vi "Multiple U3 Efunction Loop Example.vi"() -> (0 "error out 1":errorcluster)   [LabVIEW 2021]
panel:
  out "FIO5 State In 2":bool
  in  "DAC0 Voltage 2":dbl format="%.3f"
  in  "FIO4 State Out 2":bool
  out "Error Message 2":string
  out "error out 2":errorcluster
  out "AIN0 Voltage 2":dbl format="%.6f"
  in  "stop":bool
  in  "Interval (ms)":u32=500
  out "FIO5 State In 1":bool
  in  "DAC0 Voltage 1":dbl format="%.3f"
  in  "FIO4 State Out 1":bool
  out "Error Message 1":string
  out "AIN0 Voltage 1":dbl format="%.6f"
  # "U3 with LocalID=1:  Sets DAC0, sets FIO4,\nreads AIN0, and reads FIO5."
  # "U3 with LocalID=2:  Sets DAC0, sets FIO4,\nreads AIN0, and reads FIO5."
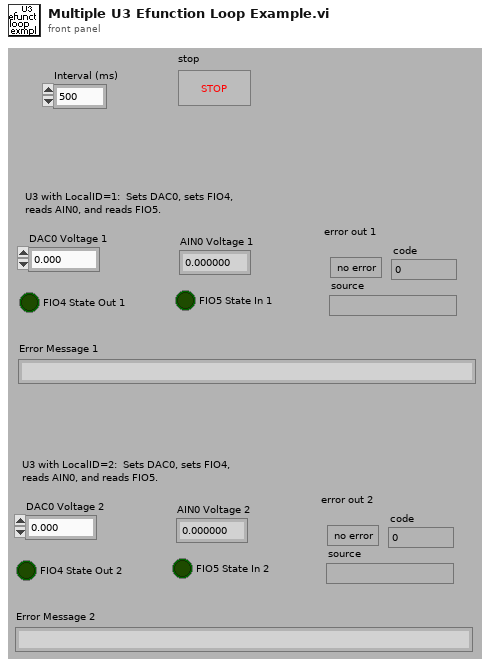
[diagram p1: front panel]
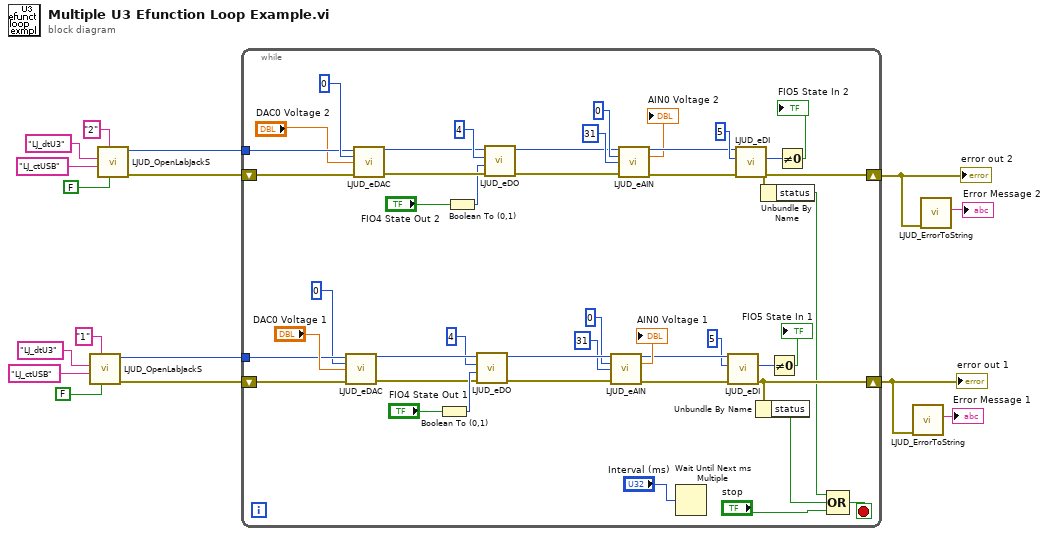
[diagram p0: block diagram]
diagram:
  n1 = call "LJUD_OpenLabJackS.vi"("FirstFound"=FALSE, "Address"="1", "ConnectionType"="LJ_ctUSB", "DeviceType"="LJ_dtU3") -> ("error out"=w11:errorcluster, "Handle"=w13:i32)  [unwired: 5 in, 1 out]
  n2 = call "LJUD_OpenLabJackS.vi"("FirstFound"=FALSE, "Address"="2", "ConnectionType"="LJ_ctUSB", "DeviceType"="LJ_dtU3") -> ("error out"=w6:errorcluster, "Handle"=w5:i32)  [unwired: 5 in, 1 out]
  n3 = while {
    shift-left: w6 -> [w40]
    shift-right: [w19] -> w1
    tunnel: w5 -> [w29]
    shift-left: w11 -> [w41]
    shift-right: [w42] -> w12
    tunnel: w13 -> [w55]
    stop <- w17 stop-if-true
    n4 = call "LJUD_eDAC.vi"("Handle In"=w55, "Channel"=0, "Voltage"="DAC0 Voltage 1", "error in"=w41) -> ("Handle Out"=w53:i32, "error out"=w54:errorcluster)  [unwired: 10 in]
    n5 = call "LJUD_eDAC.vi"("Handle In"=w29, "Channel"=0, "Voltage"="DAC0 Voltage 2", "error in"=w40) -> ("Handle Out"=w31:i32, "error out"=w30:errorcluster)  [unwired: 10 in]
    n6 = Boolean To (0,1)(Boolean="FIO4 State Out 1") -> (0, 1=w59:i16)
    n7 = Boolean To (0,1)(Boolean="FIO4 State Out 2") -> (0, 1=w27:i16)
    n8 = call "LJUD_eDO.vi"("error in"=w54, "State"=w59, "Channel"=4, "Handle In"=w53) -> ("error out"=w52:errorcluster, "Handle Out"=w51:i32)  [unwired: 6 in]
    n9 = call "LJUD_eDO.vi"("error in"=w30, "State"=w27, "Channel"=4, "Handle In"=w31) -> ("error out"=w32:errorcluster, "Handle Out"=w33:i32)  [unwired: 6 in]
    n10 = call "LJUD_eAIN.vi"("Handle In"=w51, "ChannelP"=0, "ChannelN"=31, "error in"=w52) -> ("Handle Out"=w46:i32, "Voltage"=→"AIN0 Voltage 1":dbl, "error out"=w56:errorcluster)  [unwired: 9 in]
    n11 = call "LJUD_eAIN.vi"("Handle In"=w33, "ChannelP"=0, "ChannelN"=31, "error in"=w32) -> ("Handle Out"=w38:i32, "Voltage"=→"AIN0 Voltage 2":dbl, "error out"=w28:errorcluster)  [unwired: 9 in]
    n12 = Wait Until Next ms Multiple(millisecond multiple="Interval (ms)") -> ()  [unwired: 1 out]
    n13 = call "LJUD_eDI.vi"("error in"=w56, "Channel"=5, "Handle In"=w46) -> ("error out"=w42:errorcluster, "State"=w60:i32)  [unwired: 6 in, 1 out]
    n14 = call "LJUD_eDI.vi"("error in"=w28, "Channel"=5, "Handle In"=w38) -> ("error out"=w19:errorcluster, "State"=w26:i32)  [unwired: 6 in, 1 out]
    n15 = Unbundle By Name(w42) -> ("status"=w21:bool)
    n16 = Unbundle By Name(w19) -> ("status"=w18:bool)
    n17 = Not Equal To 0?(x=w60) -> (x != 0?=→"FIO5 State In 1":bool)
    n18 = Not Equal To 0?(x=w26) -> (x != 0?=→"FIO5 State In 2":bool)
    n19 = Compound Arithmetic op=OR(w18, w21, "stop") -> (w17:bool)
  }
  "error out 1" <- w12
  "error out 2" <- w1
  n20 = call "LJUD_ErrorToString.vi"("error in"=w12) -> ("String"=→"Error Message 1":string)  [unwired: 10 in]
  n21 = call "LJUD_ErrorToString.vi"("error in"=w1) -> ("String"=→"Error Message 2":string)  [unwired: 10 in]
